vi "Create Pattern Script(Special Frames).vi"(7 "Special Frame Type":T1, 8 "error in (no error)":errorcluster, 11 "Num of Timeset":u32) -> (0 "error out":errorcluster, 3 "string out":string)   [LabVIEW 2018, in "BML_Frame_Root.lvclass"]
uses:
  BML_Frame_Root.lvclass
  Special Frame.ctl
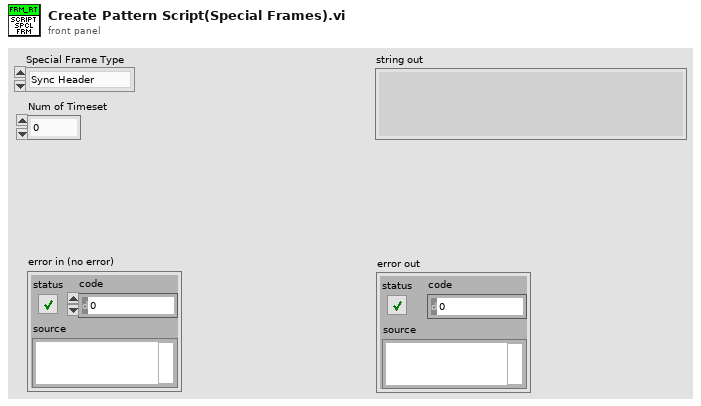
[diagram p1: front panel]
types:
  T1 = typedef "BML_Frame_Root.lvclass/Special Frame.ctl" = enum16{"Sync Header", "Protocol Header", "SW Trig", "SetID State", "Out SetID State", "SW Reset", "Wait", "SPI 4W FRM Start", "SPI 4W Wait", "SPI 4W FRM End", "SPI 4W Write Cmd", "SPI RD Collect Cmd", "SPI RD Value Cmd", "SPI 3W FRM Start", "SPI 3W Write Cmd", "SPI 3W FRM End", "SPI 3W Wait", "SPI 3W RD Cmd"}
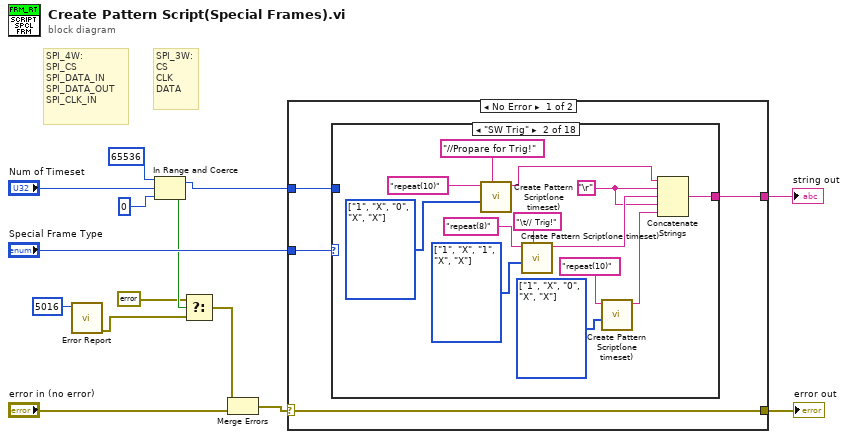
[diagram p0: block diagram]
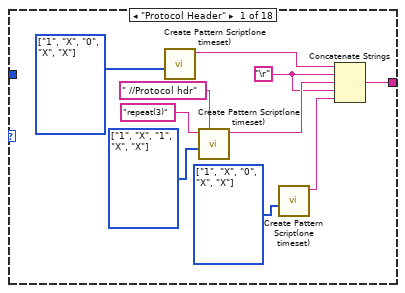
[diagram p2: hidden frame]
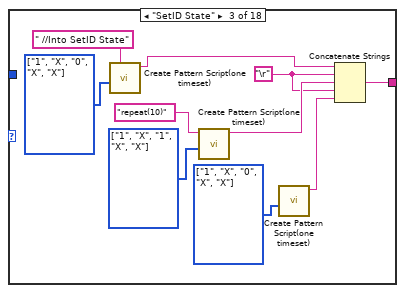
[diagram p3: hidden frame]
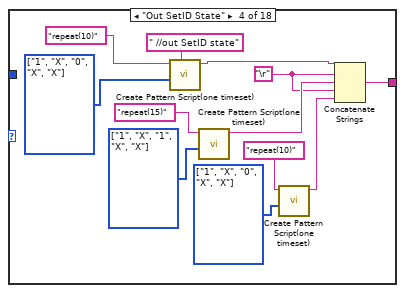
[diagram p4: hidden frame]
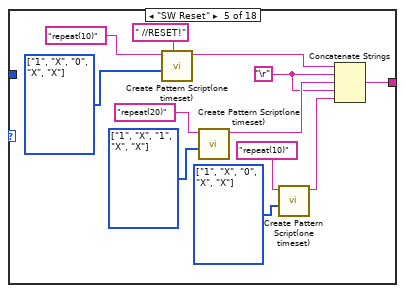
[diagram p5: hidden frame]
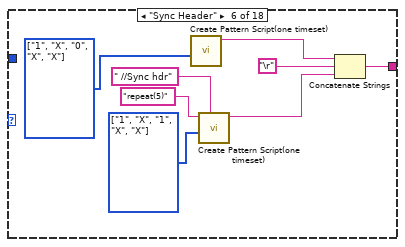
[diagram p6: hidden frame]
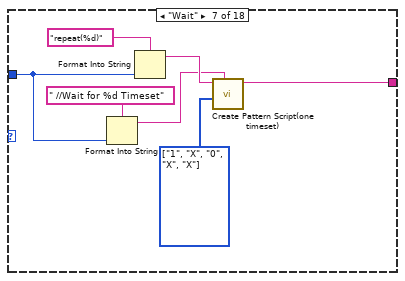
[diagram p7: hidden frame]
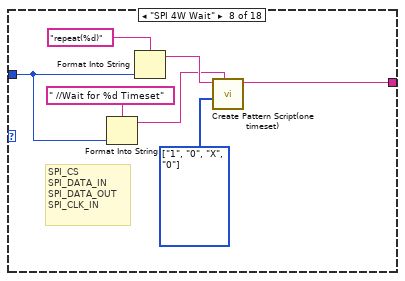
[diagram p8: hidden frame]
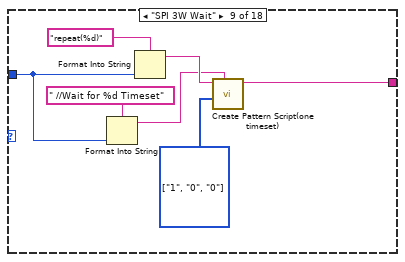
[diagram p9: hidden frame]
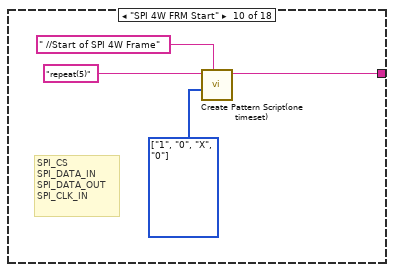
[diagram p10: hidden frame]
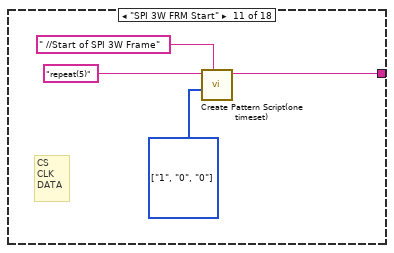
[diagram p11: hidden frame]
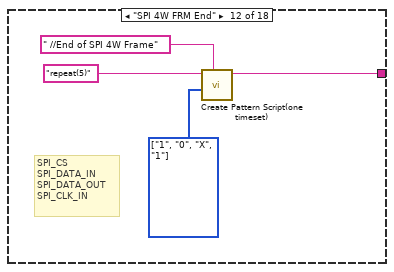
[diagram p12: hidden frame]
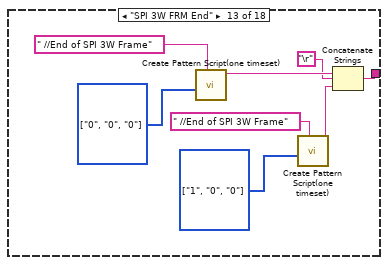
[diagram p13: hidden frame]
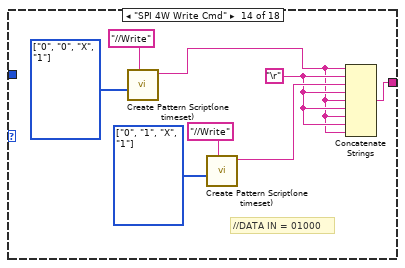
[diagram p14: hidden frame]
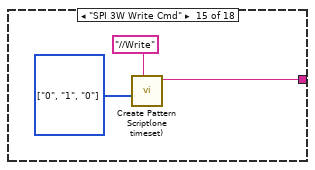
[diagram p15: hidden frame]
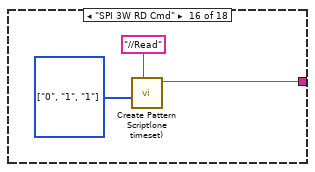
[diagram p16: hidden frame]
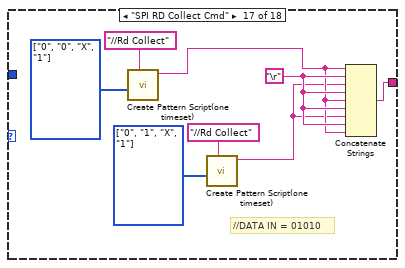
[diagram p17: hidden frame]
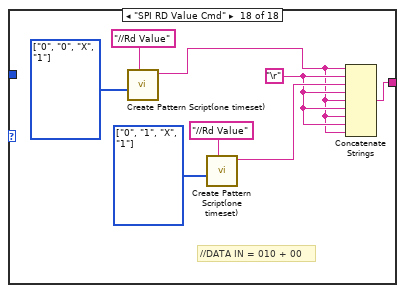
[diagram p18: hidden frame]
diagram:
  # "SPI_3W:\nCS\nCLK\nDATA"
  # "SPI_4W:\nSPI_CS\nSPI_DATA_IN\nSPI_DATA_OUT\nSPI_CLK_IN"
  n1 = call "Error Report.vi"("Error Code"=i16 5016) -> ("error out"=w4:errorcluster)  [unwired: 10 in]
  n2 = In Range and Coerce(upper limit=u32 65536, x="Num of Timeset", lower limit=u32 0) -> (coerced(x)=w8:u32, In Range?=w7:bool)
  n3 = Select(t=errorcluster {"status"=FALSE, "code"=0, "source"=""} ("error in (no error)"), s=w7, f=w4) -> (s? t:f=w3:errorcluster)
  n4 = Merge Errors(w3, "error in (no error)") -> (w1:errorcluster)
  n5 = case shown="No Error" w1 {
    selector: w1 -> [w15 w155]
    tunnel: [w15 w155] -> w14
    tunnel: "Special Frame Type" -> [w18 _]
    tunnel: [w17 _] -> w12
    tunnel: w8 -> [w16 _]
    frame No Error {
      n6 = case shown="\"SW Trig\"" w18 {
        tunnel: [w21 w34 w44 w56 w68 w78 w84 w91 w98 w107 w111 w115 w119 w125 w133 w136 w140 w150] -> w17
        tunnel: w16 -> [_ _ _ _ _ _ w87 w94 w101 _ _ _ _ _ _ _ _ _]
        frame "Protocol Header" {
          w22 = "\r"
          w25 = enum16{"0", "1", "L", "H", "X", "V", "D", "M"}[] [enum."1", enum."X", enum."0", enum."X", enum."X"] items=["0", "1", "L", "H", "X", "V", "D", "M"] ("PinState")
          w27 = enum16{"0", "1", "L", "H", "X", "V", "D", "M"}[] [enum."1", enum."X", enum."1", enum."X", enum."X"] items=["0", "1", "L", "H", "X", "V", "D", "M"] ("PinState")
          w28 = enum16{"0", "1", "L", "H", "X", "V", "D", "M"}[] [enum."1", enum."X", enum."0", enum."X", enum."X"] items=["0", "1", "L", "H", "X", "V", "D", "M"] ("PinState")
          n7 = call "Create Pattern Script(one timeset).vi"("PinState"=w28) -> ("string out"=w20:string)  [unwired: 10 in]
          n8 = call "Create Pattern Script(one timeset).vi"("Notes"=" //Protocol hdr" ("string"), "PinState"=w27, "opcode"="repeat(3)") -> ("string out"=w24:string)  [unwired: 8 in]
          n9 = call "Create Pattern Script(one timeset).vi"("PinState"=w25) -> ("string out"=w23:string)  [unwired: 10 in]
          n10 = Concatenate Strings(w20, w22, w24, w22, w23) -> (w21:string)
        }
        frame "SW Trig" {
          w35 = "\r"
          w38 = enum16{"0", "1", "L", "H", "X", "V", "D", "M"}[] [enum."1", enum."X", enum."0", enum."X", enum."X"] items=["0", "1", "L", "H", "X", "V", "D", "M"] ("PinState")
          w40 = enum16{"0", "1", "L", "H", "X", "V", "D", "M"}[] [enum."1", enum."X", enum."1", enum."X", enum."X"] items=["0", "1", "L", "H", "X", "V", "D", "M"] ("PinState")
          w41 = enum16{"0", "1", "L", "H", "X", "V", "D", "M"}[] [enum."1", enum."X", enum."0", enum."X", enum."X"] items=["0", "1", "L", "H", "X", "V", "D", "M"] ("PinState")
          n11 = call "Create Pattern Script(one timeset).vi"("Notes"="//Propare for Trig!", "PinState"=w41, "opcode"="repeat(10)") -> ("string out"=w30:string)  [unwired: 8 in]
          n12 = call "Create Pattern Script(one timeset).vi"("Notes"="\t// Trig!", "PinState"=w40, "opcode"="repeat(8)") -> ("string out"=w37:string)  [unwired: 8 in]
          n13 = call "Create Pattern Script(one timeset).vi"("PinState"=w38, "opcode"="repeat(10)") -> ("string out"=w36:string)  [unwired: 9 in]
          n14 = Concatenate Strings(w30, w35, w37, w35, w36) -> (w34:string)
        }
        frame "SetID State" {
          w45 = "\r"
          w48 = enum16{"0", "1", "L", "H", "X", "V", "D", "M"}[] [enum."1", enum."X", enum."0", enum."X", enum."X"] items=["0", "1", "L", "H", "X", "V", "D", "M"] ("PinState")
          w50 = enum16{"0", "1", "L", "H", "X", "V", "D", "M"}[] [enum."1", enum."X", enum."1", enum."X", enum."X"] items=["0", "1", "L", "H", "X", "V", "D", "M"] ("PinState")
          w51 = enum16{"0", "1", "L", "H", "X", "V", "D", "M"}[] [enum."1", enum."X", enum."0", enum."X", enum."X"] items=["0", "1", "L", "H", "X", "V", "D", "M"] ("PinState")
          n15 = call "Create Pattern Script(one timeset).vi"("Notes"=" //Into SetID State" ("string"), "PinState"=w51) -> ("string out"=w42:string)  [unwired: 9 in]
          n16 = call "Create Pattern Script(one timeset).vi"("PinState"=w50, "opcode"="repeat(10)") -> ("string out"=w47:string)  [unwired: 9 in]
          n17 = call "Create Pattern Script(one timeset).vi"("PinState"=w48) -> ("string out"=w46:string)  [unwired: 10 in]
          n18 = Concatenate Strings(w42, w45, w47, w45, w46) -> (w44:string)
        }
        frame "Out SetID State" {
          w57 = "\r"
          w60 = enum16{"0", "1", "L", "H", "X", "V", "D", "M"}[] [enum."1", enum."X", enum."0", enum."X", enum."X"] items=["0", "1", "L", "H", "X", "V", "D", "M"] ("PinState")
          w62 = enum16{"0", "1", "L", "H", "X", "V", "D", "M"}[] [enum."1", enum."X", enum."1", enum."X", enum."X"] items=["0", "1", "L", "H", "X", "V", "D", "M"] ("PinState")
          w63 = enum16{"0", "1", "L", "H", "X", "V", "D", "M"}[] [enum."1", enum."X", enum."0", enum."X", enum."X"] items=["0", "1", "L", "H", "X", "V", "D", "M"] ("PinState")
          n19 = call "Create Pattern Script(one timeset).vi"("Notes"=" //out SetID state" ("string"), "PinState"=w63, "opcode"="repeat(10)") -> ("string out"=w52:string)  [unwired: 8 in]
          n20 = call "Create Pattern Script(one timeset).vi"("PinState"=w62, "opcode"="repeat(15)") -> ("string out"=w59:string)  [unwired: 9 in]
          n21 = call "Create Pattern Script(one timeset).vi"("PinState"=w60, "opcode"="repeat(10)") -> ("string out"=w58:string)  [unwired: 9 in]
          n22 = Concatenate Strings(w52, w57, w59, w57, w58) -> (w56:string)
        }
        frame "SW Reset" {
          w69 = "\r"
          w72 = enum16{"0", "1", "L", "H", "X", "V", "D", "M"}[] [enum."1", enum."X", enum."0", enum."X", enum."X"] items=["0", "1", "L", "H", "X", "V", "D", "M"] ("PinState")
          w74 = enum16{"0", "1", "L", "H", "X", "V", "D", "M"}[] [enum."1", enum."X", enum."1", enum."X", enum."X"] items=["0", "1", "L", "H", "X", "V", "D", "M"] ("PinState")
          w75 = enum16{"0", "1", "L", "H", "X", "V", "D", "M"}[] [enum."1", enum."X", enum."0", enum."X", enum."X"] items=["0", "1", "L", "H", "X", "V", "D", "M"] ("PinState")
          n23 = call "Create Pattern Script(one timeset).vi"("Notes"=" //RESET!" ("string"), "PinState"=w75, "opcode"="repeat(10)") -> ("string out"=w65:string)  [unwired: 8 in]
          n24 = call "Create Pattern Script(one timeset).vi"("PinState"=w74, "opcode"="repeat(20)") -> ("string out"=w71:string)  [unwired: 9 in]
          n25 = call "Create Pattern Script(one timeset).vi"("PinState"=w72, "opcode"="repeat(10)") -> ("string out"=w70:string)  [unwired: 9 in]
          n26 = Concatenate Strings(w65, w69, w71, w69, w70) -> (w68:string)
        }
        frame "Sync Header" {
          w82 = enum16{"0", "1", "L", "H", "X", "V", "D", "M"}[] [enum."1", enum."X", enum."1", enum."X", enum."X"] items=["0", "1", "L", "H", "X", "V", "D", "M"] ("PinState")
          w83 = enum16{"0", "1", "L", "H", "X", "V", "D", "M"}[] [enum."1", enum."X", enum."0", enum."X", enum."X"] items=["0", "1", "L", "H", "X", "V", "D", "M"] ("PinState")
          n27 = call "Create Pattern Script(one timeset).vi"("PinState"=w83) -> ("string out"=w77:string)  [unwired: 10 in]
          n28 = call "Create Pattern Script(one timeset).vi"("Notes"=" //Sync hdr" ("string"), "PinState"=w82, "opcode"="repeat(5)") -> ("string out"=w80:string)  [unwired: 8 in]
          n29 = Concatenate Strings(w77, "\r", w80) -> (w78:string)
        }
        frame "Wait" {
          w90 = enum16{"0", "1", "L", "H", "X", "V", "D", "M"}[] [enum."1", enum."X", enum."0", enum."X", enum."X"] items=["0", "1", "L", "H", "X", "V", "D", "M"] ("PinState")
          n30 = Format Into String(format string=" //Wait for %d Timeset", w87) -> (resulting string=w85:string)  [unwired: 2 in, 1 out]
          n31 = Format Into String(format string="repeat(%d)", w87) -> (resulting string=w88:string)  [unwired: 2 in, 1 out]
          n32 = call "Create Pattern Script(one timeset).vi"("Notes"=w85, "PinState"=w90, "opcode"=w88) -> ("string out"=w84:string)  [unwired: 8 in]
        }
        frame "SPI 4W Wait" {
          w97 = enum16{"0", "1", "L", "H", "X", "V", "D", "M"}[] [enum."1", enum."0", enum."X", enum."0"] items=["0", "1", "L", "H", "X", "V", "D", "M"] ("PinState")
          # "SPI_CS\nSPI_DATA_IN\nSPI_DATA_OUT\nSPI_CLK_IN"
          n33 = Format Into String(format string=" //Wait for %d Timeset", w94) -> (resulting string=w92:string)  [unwired: 2 in, 1 out]
          n34 = Format Into String(format string="repeat(%d)", w94) -> (resulting string=w95:string)  [unwired: 2 in, 1 out]
          n35 = call "Create Pattern Script(one timeset).vi"("Notes"=w92, "PinState"=w97, "opcode"=w95) -> ("string out"=w91:string)  [unwired: 8 in]
        }
        frame "SPI 3W Wait" {
          w104 = enum16{"0", "1", "L", "H", "X", "V", "D", "M"}[] [enum."1", enum."0", enum."0"] items=["0", "1", "L", "H", "X", "V", "D", "M"] ("PinState")
          n36 = Format Into String(format string=" //Wait for %d Timeset", w101) -> (resulting string=w99:string)  [unwired: 2 in, 1 out]
          n37 = Format Into String(format string="repeat(%d)", w101) -> (resulting string=w102:string)  [unwired: 2 in, 1 out]
          n38 = call "Create Pattern Script(one timeset).vi"("Notes"=w99, "PinState"=w104, "opcode"=w102) -> ("string out"=w98:string)  [unwired: 8 in]
        }
        frame "SPI 4W FRM Start" {
          w108 = enum16{"0", "1", "L", "H", "X", "V", "D", "M"}[] [enum."1", enum."0", enum."X", enum."0"] items=["0", "1", "L", "H", "X", "V", "D", "M"] ("PinState")
          # "SPI_CS\nSPI_DATA_IN\nSPI_DATA_OUT\nSPI_CLK_IN"
          n39 = call "Create Pattern Script(one timeset).vi"("Notes"=" //Start of SPI 4W Frame" ("format string"), "PinState"=w108, "opcode"="repeat(5)" ("format string")) -> ("string out"=w107:string)  [unwired: 8 in]
        }
        frame "SPI 3W FRM Start" {
          w112 = enum16{"0", "1", "L", "H", "X", "V", "D", "M"}[] [enum."1", enum."0", enum."0"] items=["0", "1", "L", "H", "X", "V", "D", "M"] ("PinState")
          # "CS\nCLK\nDATA"
          n40 = call "Create Pattern Script(one timeset).vi"("Notes"=" //Start of SPI 3W Frame" ("format string"), "PinState"=w112, "opcode"="repeat(5)" ("format string")) -> ("string out"=w111:string)  [unwired: 8 in]
        }
        frame "SPI 4W FRM End" {
          w116 = enum16{"0", "1", "L", "H", "X", "V", "D", "M"}[] [enum."1", enum."0", enum."X", enum."1"] items=["0", "1", "L", "H", "X", "V", "D", "M"] ("PinState")
          # "SPI_CS\nSPI_DATA_IN\nSPI_DATA_OUT\nSPI_CLK_IN"
          n41 = call "Create Pattern Script(one timeset).vi"("Notes"=" //End of SPI 4W Frame" ("format string"), "PinState"=w116, "opcode"="repeat(5)" ("format string")) -> ("string out"=w115:string)  [unwired: 8 in]
        }
        frame "SPI 3W FRM End" {
          w122 = enum16{"0", "1", "L", "H", "X", "V", "D", "M"}[] [enum."1", enum."0", enum."0"] items=["0", "1", "L", "H", "X", "V", "D", "M"] ("PinState")
          w124 = enum16{"0", "1", "L", "H", "X", "V", "D", "M"}[] [enum."0", enum."0", enum."0"] items=["0", "1", "L", "H", "X", "V", "D", "M"] ("PinState")
          n42 = call "Create Pattern Script(one timeset).vi"("Notes"=" //End of SPI 3W Frame" ("format string"), "PinState"=w124) -> ("string out"=w120:string)  [unwired: 9 in]
          n43 = call "Create Pattern Script(one timeset).vi"("Notes"=" //End of SPI 3W Frame" ("format string"), "PinState"=w122) -> ("string out"=w117:string)  [unwired: 9 in]
          n44 = Concatenate Strings(w120, "\r", w117) -> (w119:string)
        }
        frame "SPI 4W Write Cmd" {
          w131 = enum16{"0", "1", "L", "H", "X", "V", "D", "M"}[] [enum."0", enum."1", enum."X", enum."1"] items=["0", "1", "L", "H", "X", "V", "D", "M"] ("PinState")
          w127 = "\r"
          w132 = enum16{"0", "1", "L", "H", "X", "V", "D", "M"}[] [enum."0", enum."0", enum."X", enum."1"] items=["0", "1", "L", "H", "X", "V", "D", "M"] ("PinState")
          # "//DATA IN = 01000"
          n45 = call "Create Pattern Script(one timeset).vi"("Notes"="//Write", "PinState"=w132) -> ("string out"=w126:string)  [unwired: 9 in]
          n46 = call "Create Pattern Script(one timeset).vi"("Notes"="//Write", "PinState"=w131) -> ("string out"=w128:string)  [unwired: 9 in]
          n47 = Concatenate Strings(w126, w127, w128, w127, w126, w127, w126, w127, w126) -> (w125:string)
        }
        frame "SPI 3W Write Cmd" {
          w135 = enum16{"0", "1", "L", "H", "X", "V", "D", "M"}[] [enum."0", enum."1", enum."0"] items=["0", "1", "L", "H", "X", "V", "D", "M"] ("PinState")
          n48 = call "Create Pattern Script(one timeset).vi"("Notes"="//Write", "PinState"=w135) -> ("string out"=w133:string)  [unwired: 9 in]
        }
        frame "SPI 3W RD Cmd" {
          w138 = enum16{"0", "1", "L", "H", "X", "V", "D", "M"}[] [enum."0", enum."1", enum."1"] items=["0", "1", "L", "H", "X", "V", "D", "M"] ("PinState")
          n49 = call "Create Pattern Script(one timeset).vi"("Notes"="//Read", "PinState"=w138) -> ("string out"=w136:string)  [unwired: 9 in]
        }
        frame "SPI RD Collect Cmd" {
          w145 = enum16{"0", "1", "L", "H", "X", "V", "D", "M"}[] [enum."0", enum."1", enum."X", enum."1"] items=["0", "1", "L", "H", "X", "V", "D", "M"] ("PinState")
          w142 = "\r"
          w146 = enum16{"0", "1", "L", "H", "X", "V", "D", "M"}[] [enum."0", enum."0", enum."X", enum."1"] items=["0", "1", "L", "H", "X", "V", "D", "M"] ("PinState")
          # "//DATA IN = 01010"
          n50 = call "Create Pattern Script(one timeset).vi"("Notes"="//Rd Collect", "PinState"=w146) -> ("string out"=w141:string)  [unwired: 9 in]
          n51 = call "Create Pattern Script(one timeset).vi"("Notes"="//Rd Collect", "PinState"=w145) -> ("string out"=w139:string)  [unwired: 9 in]
          n52 = Concatenate Strings(w141, w142, w139, w142, w141, w142, w139, w142, w141) -> (w140:string)
        }
        frame "SPI RD Value Cmd" {
          w153 = enum16{"0", "1", "L", "H", "X", "V", "D", "M"}[] [enum."0", enum."1", enum."X", enum."1"] items=["0", "1", "L", "H", "X", "V", "D", "M"] ("PinState")
          w148 = "\r"
          w154 = enum16{"0", "1", "L", "H", "X", "V", "D", "M"}[] [enum."0", enum."0", enum."X", enum."1"] items=["0", "1", "L", "H", "X", "V", "D", "M"] ("PinState")
          # "//DATA IN = 010 + 00"
          n53 = call "Create Pattern Script(one timeset).vi"("Notes"="//Rd Value", "PinState"=w154) -> ("string out"=w147:string)  [unwired: 9 in]
          n54 = call "Create Pattern Script(one timeset).vi"("Notes"="//Rd Value", "PinState"=w153) -> ("string out"=w149:string)  [unwired: 9 in]
          n55 = Concatenate Strings(w147, w148, w149, w148, w147, w148, w147, w148, w147) -> (w150:string)
        }
      }
    }
    frame Error {
    }
  }
  "error out" <- w14
  "string out" <- w12
